vi "Configure.vi"(7 "Enum":enum16{"Read", "Write"}(ring), 11 "Port 4":refnum<vi>) -> (3 "Port 5":refnum<vi>)   [LabVIEW 2013]
uses:
  Control/Port.ctl
  Control/Buffer.vi
  <vilib>/Utility/config.llb/Read Key (String).vi
  <vilib>/Utility/config.llb/Read Key (I32).vi
  <vilib>/Utility/config.llb/Write Key (String).vi
  <vilib>/Utility/config.llb/NI_LVConfig.lvlib
panel:
  out "Boolean":bool
  out "s? t:f":string
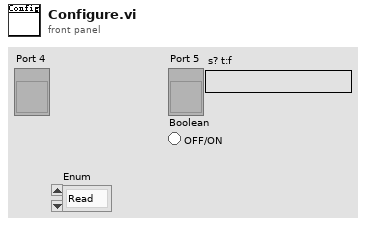
[diagram p1: front panel]
types:
  T1 = typedef "NI_LVConfig.lvlib/Config Data RefNum.ctl" = refnum<k1>
  T2 = typedef "Port.ctl" = cluster{"Multimeter":refnum<visa-resource-name>, "ACsource ":refnum<visa-resource-name>, "GEA":refnum<visa-resource-name>, "WT200":refnum<visa-resource-name>, "AutoScan":refnum<visa-resource-name>, "lines":tag, "MabeCOM":refnum<visa-resource-name>}
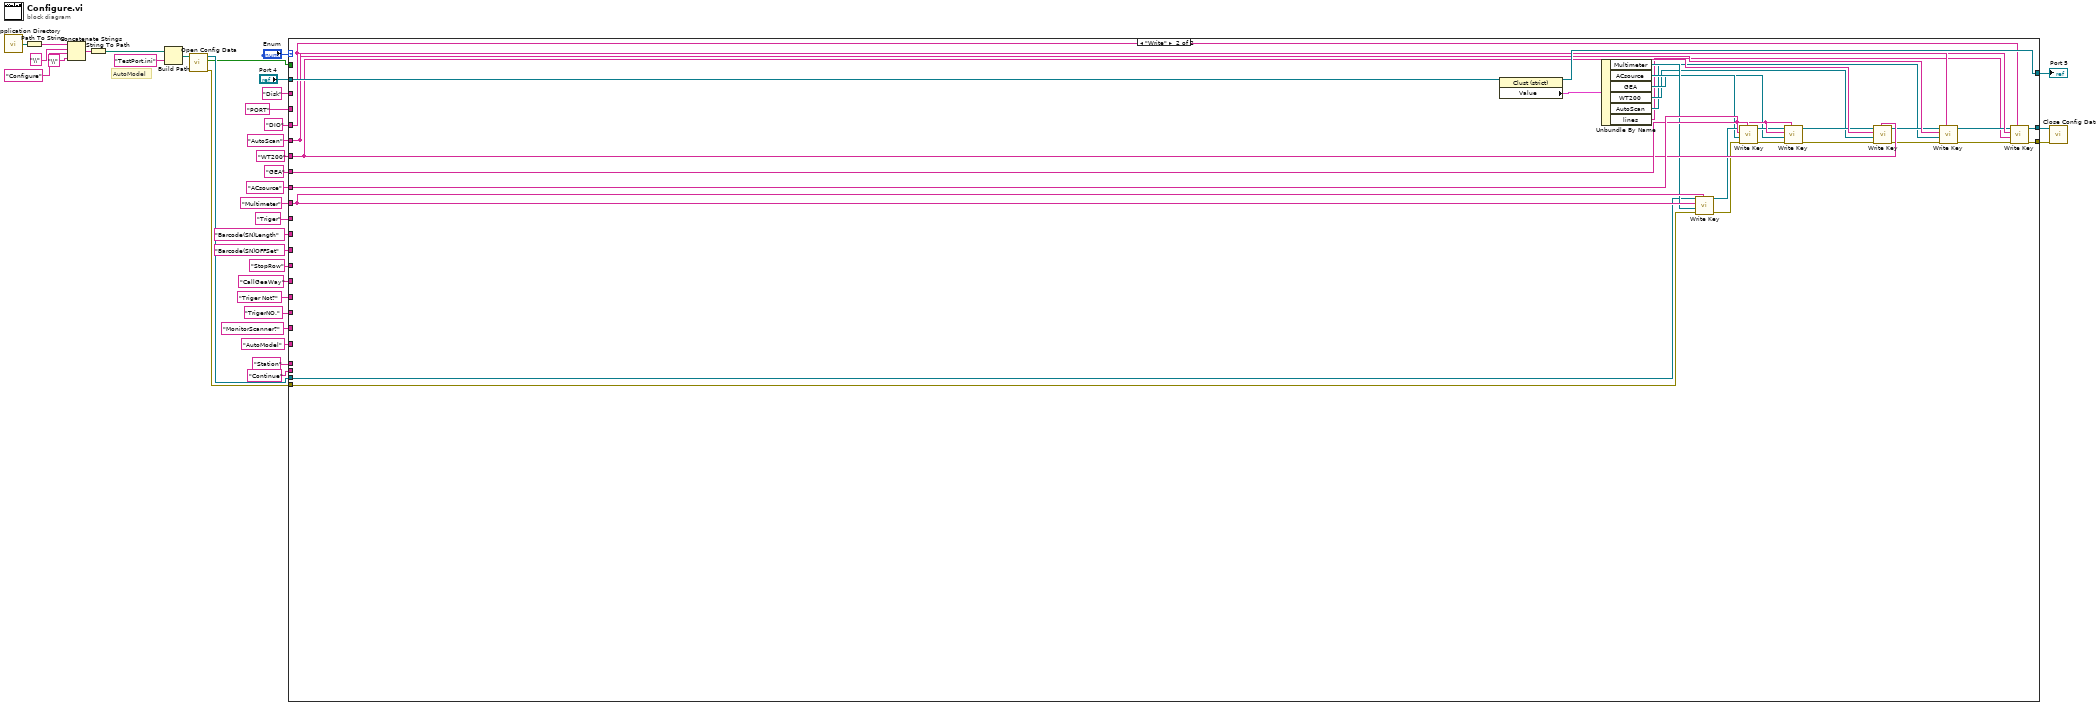
[diagram p0: block diagram]
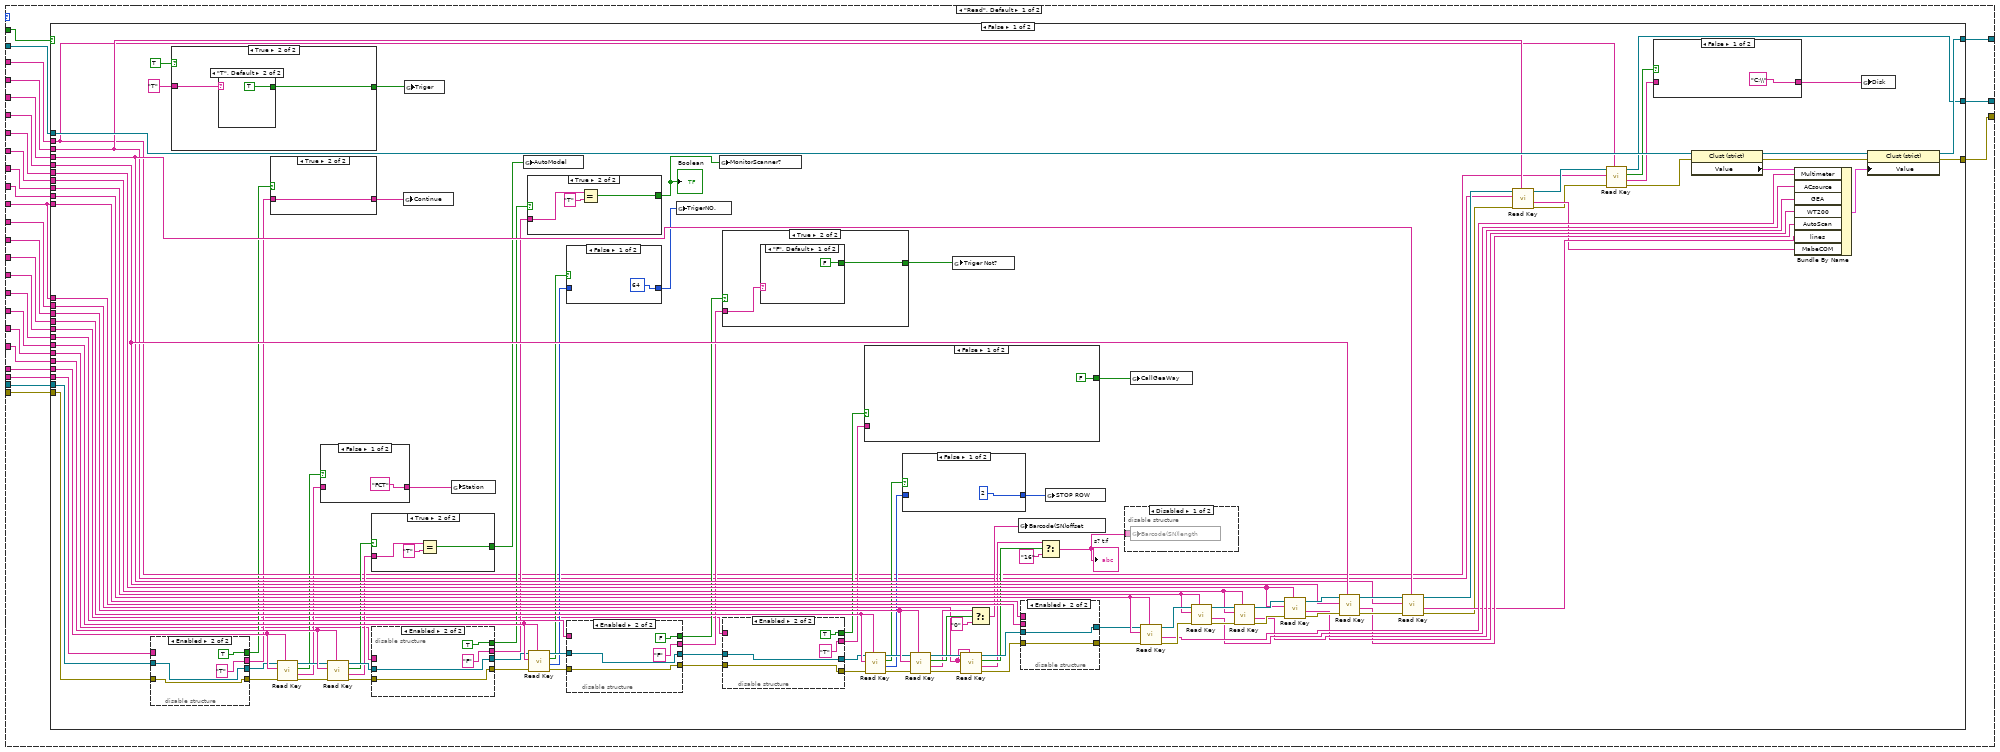
[diagram p2: hidden frame]
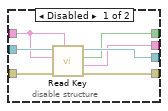
[diagram p4: hidden frame]
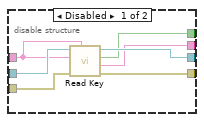
[diagram p5: hidden frame]
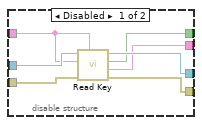
[diagram p6: hidden frame]
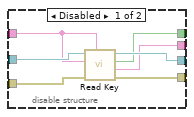
[diagram p7: hidden frame]
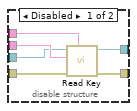
[diagram p8: hidden frame]
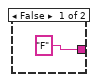
[diagram p9: hidden frame]
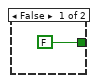
[diagram p12: hidden frame]
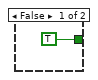
[diagram p13: hidden frame]
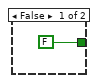
[diagram p14: hidden frame]
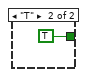
[diagram p15: hidden frame]
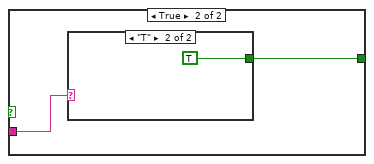
[diagram p17: hidden frame]
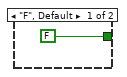
[diagram p18: hidden frame]
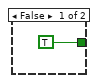
[diagram p20: hidden frame]
diagram:
  # "AutoModel"
  n1 = call <vilib>:"Application Directory.vi"() -> ("Application Directory"=w22:path)
  n2 = Path To String(path=w22) -> (string=w21:string)
  n3 = Concatenate Strings(w21, "\\" ("string"), "Configure" ("string"), "\\" ("string")) -> (w18:string)
  n4 = String To Path(string=w18) -> (path=w16:path)
  n5 = Build Path(base path=w16, name or relative path="TestPort.ini") -> (appended path=w34:path)
  n6 = call <vilib>:"Open Config Data.vi"("configuration file path"=w34) -> ("error out"=w32:errorcluster, "file created?"=w23:bool, "refnum"=w33:T1)  [unwired: 8 in]
  n7 = case shown="\"Write\"" "Enum" {
    tunnel: "Port 4" -> [w59 w292]
    tunnel: [w62 w291] -> w5
    tunnel: w33 -> [w61 w265]
    tunnel: w32 -> [w60 w264]
    tunnel: "Multimeter" ("section") -> [w56 w289]
    tunnel: "ACsource" ("section") -> [w55 w288]
    tunnel: "GEA" ("section") -> [w54 w287]
    tunnel: "WT200" ("section") -> [w53 w286]
    tunnel: "AutoScan" ("section") -> [w52 w285]
    tunnel: "DIO" ("section") -> [w51 w284]
    tunnel: [w57 w267] -> w25
    tunnel: [w58 w266] -> w24
    tunnel: w23 -> [w50 _]
    tunnel: "Triger" ("section") -> [w39 _]
    tunnel: "Barcode(SN)OFFSet" -> [w49 _]
    tunnel: "Barcode(SN)Length" -> [w37 _]
    tunnel: "StopRow" -> [w48 _]
    tunnel: "CallGeaWay" -> [w47 _]
    tunnel: "TrigerNO." -> [w46 _]
    tunnel: "Triger Not?" -> [w45 _]
    tunnel: "MonitorScanner?" ("section") -> [w38 _]
    tunnel: "AutoModel" -> [w44 _]
    tunnel: "PORT" -> [w43 _]
    tunnel: "Disk" -> [w42 _]
    tunnel: "Station" -> [w41 _]
    tunnel: "Continue" -> [w40 _]
    frame "Read", Default {
      n8 = case shown="False" w50 {
        tunnel: [w174 w263] -> w62
        tunnel: w61 -> [w72 w262]
        tunnel: w60 -> [w70 w261]
        tunnel: w59 -> [w173 w263]
        tunnel: [w148 w261] -> w58
        tunnel: [w85 w262] -> w57
        tunnel: w56 -> [w161 _]
        tunnel: w55 -> [w160 _]
        tunnel: w54 -> [w159 _]
        tunnel: w53 -> [w158 _]
        tunnel: w52 -> [w157 _]
        tunnel: w51 -> [w156 _]
        tunnel: w39 -> [w147 _]
        tunnel: w39 -> [w146 _]
        tunnel: w49 -> [w128 _]
        tunnel: w37 -> [w127 _]
        tunnel: w48 -> [w124 _]
        tunnel: w47 -> [w65 _]
        tunnel: w46 -> [w115 _]
        tunnel: w45 -> [w110 _]
        tunnel: w38 -> [w64 _]
        tunnel: w44 -> [w97 _]
        tunnel: w43 -> [w87 _]
        tunnel: w42 -> [w82 _]
        tunnel: w41 -> [w76 _]
        tunnel: w40 -> [w63 _]
        frame False {
          n9 = disable-structure shown="Enabled" {
            disable-tunnel: w72 -> [w182 w185]
            disable-tunnel: [w181 w185] -> w71
            disable-tunnel: w70 -> [w180 w186]
            disable-tunnel: [w179 w186] -> w69
            disable-tunnel: [w178 TRUE ("found?")] -> w68
            disable-tunnel: [w177 "T"] -> w67
            disable-tunnel: w63 -> [w176 _]
            frame Disabled {
              n10 = call-poly <vilib>:"Read Key.vi"("section"=w176, "error in (no error)"=w180, "key"=w176, "refnum"=w182) -> ("error out"=w179:errorcluster, "value"=w177:string, "found?"=w178:bool, "refnum out"=w181:T1)  [unwired: 4 in]
            }
            frame Enabled {
            }
          }
          n11 = case shown="True" TRUE ("found?") {
            tunnel: "T" ("value") -> [_ w258]
            tunnel: [TRUE w257] -> w141
            frame False {
            }
            frame True {
              n12 = case shown="\"T\", Default" w258 {
                tunnel: [FALSE TRUE] -> w257
                frame "F" {
                }
                frame "T", Default {
                }
              }
            }
          }
          n13 = case shown="True" w68 {
            tunnel: w67 -> [_ w229]
            tunnel: ["F" ("value") w229] -> w66
            frame False {
            }
            frame True {
            }
          }
          n14 = call-poly <vilib>:"Read Key.vi"("section"=w76, "error in (no error)"=w69, "key"=w76, "refnum"=w71) -> ("error out"=w77:errorcluster, "value"=w75:string, "found?"=w74:bool, "refnum out"=w78:T1)  [unwired: 4 in]
          n15 = case shown="False" w74 {
            tunnel: w75 -> [_ w231]
            tunnel: ["FCT" ("value") w231] -> w73
            frame False {
            }
            frame True {
            }
          }
          n16 = call-poly <vilib>:"Read Key.vi"("section"=w97, "error in (no error)"=w77, "key"=w97, "refnum"=w78) -> ("error out"=w95:errorcluster, "value"=w94:string, "found?"=w93:bool, "refnum out"=w96:T1)  [unwired: 4 in]
          n17 = case shown="True" w93 {
            tunnel: [FALSE w235] -> w98
            tunnel: w94 -> [_ w237]
            frame False {
            }
            frame True {
              n18 = Equal?(x=w237, y="T") -> (x = y?=w235:bool)
            }
          }
          n19 = disable-structure shown="Enabled" {
            disable-tunnel: [w193 w196] -> w103
            disable-tunnel: [w192 w197] -> w102
            disable-tunnel: [w191 "F"] -> w100
            disable-tunnel: [w190 TRUE ("found?")] -> w99
            disable-tunnel: w96 -> [w189 w196]
            disable-tunnel: w95 -> [w188 w197]
            disable-tunnel: w64 -> [w187 _]
            frame Disabled {
              n20 = call-poly <vilib>:"Read Key.vi"("section"=w187, "error in (no error)"=w188, "key"=w187, "refnum"=w189) -> ("error out"=w192:errorcluster, "value"=w191:string, "found?"=w190:bool, "refnum out"=w193:T1)  [unwired: 4 in]
            }
            frame Enabled {
            }
          }
          n21 = global write "Buffer.vi" "Continue"(w66) -> ()
          n22 = global write "Buffer.vi" "Triger"(w141) -> ()
          n23 = global write "Buffer.vi" "Station"(w73) -> ()
          n24 = global write "Buffer.vi" "AutoModel"(w98) -> ()
          n25 = case shown="True" w99 {
            tunnel: [TRUE w239] -> w101
            tunnel: w100 -> [_ w241]
            frame False {
            }
            frame True {
              n26 = Equal?(x=w241, y="T") -> (x = y?=w239:bool)
            }
          }
          "Boolean" <- w101
          n27 = call-poly <vilib>:"Read Key.vi"("section"=w115, "error in (no error)"=w102, "key"=w115, "refnum"=w103) -> ("error out"=w114:errorcluster, "value"=w108:i32, "found?"=w109:bool, "refnum out"=w113:T1)  [unwired: 4 in]
          n28 = case shown="False" w109 {
            tunnel: w108 -> [_ w248]
            tunnel: [64 ("value") w248] -> w107
            frame False {
            }
            frame True {
            }
          }
          n29 = disable-structure shown="Enabled" {
            disable-tunnel: w114 -> [w215 w219]
            disable-tunnel: w113 -> [w214 w218]
            disable-tunnel: [w213 w218] -> w112
            disable-tunnel: [w212 w219] -> w111
            disable-tunnel: w110 -> [w211 _]
            disable-tunnel: [w210 FALSE] -> w106
            disable-tunnel: [w209 "F"] -> w105
            frame Disabled {
              n30 = call-poly <vilib>:"Read Key.vi"("section"=w211, "error in (no error)"=w215, "key"=w211, "refnum"=w214) -> ("error out"=w212:errorcluster, "value"=w209:string, "found?"=w210:bool, "refnum out"=w213:T1)  [unwired: 4 in]
            }
            frame Enabled {
            }
          }
          n31 = global write "Buffer.vi" "TrigerNO."(w107) -> ()
          n32 = global write "Buffer.vi" "MonitorScanner?"(w101) -> ()
          n33 = case shown="True" w106 {
            tunnel: w105 -> [_ w244]
            tunnel: [FALSE ("value") w243] -> w104
            frame False {
            }
            frame True {
              n34 = case shown="\"F\", Default" w244 {
                tunnel: [FALSE TRUE] -> w243
                frame "F", Default {
                }
                frame "T" {
                }
              }
            }
          }
          n35 = disable-structure shown="Enabled" {
            disable-tunnel: [w204 w207] -> w120
            disable-tunnel: [w203 w208] -> w119
            disable-tunnel: [w202 "T"] -> w118
            disable-tunnel: [w201 TRUE] -> w116
            disable-tunnel: w112 -> [w200 w207]
            disable-tunnel: w111 -> [w199 w208]
            disable-tunnel: w65 -> [w198 _]
            frame Disabled {
              n36 = call-poly <vilib>:"Read Key.vi"("section"=w198, "error in (no error)"=w199, "key"=w198, "refnum"=w200) -> ("error out"=w203:errorcluster, "value"=w202:string, "found?"=w201:bool, "refnum out"=w204:T1)  [unwired: 4 in]
            }
            frame Enabled {
            }
          }
          n37 = case shown="False" w116 {
            tunnel: w118 -> [_ w251]
            tunnel: [FALSE w250] -> w117
            frame False {
            }
            frame True {
              n38 = case shown="\"T\"" w251 {
                tunnel: [FALSE TRUE] -> w250
                frame "F", Default {
                }
                frame "T" {
                }
              }
            }
          }
          n39 = call-poly <vilib>:"Read Key.vi"("section"=w124, "error in (no error)"=w119, "key"=w124, "refnum"=w120) -> ("error out"=w125:errorcluster, "value"=w122:i32, "found?"=w123:bool, "refnum out"=w126:T1)  [unwired: 4 in]
          n40 = case shown="False" w123 {
            tunnel: w122 -> [_ w255]
            tunnel: [2 ("value") w255] -> w121
            frame False {
            }
            frame True {
            }
          }
          n41 = call-poly <vilib>:"Read Key.vi"("section"=w128, "error in (no error)"=w125, "key"=w128, "refnum"=w126) -> ("error out"=w138:errorcluster, "value"=w134:string, "found?"=w136:bool, "refnum out"=w140:T1)  [unwired: 4 in]
          n42 = global write "Buffer.vi" "Triger Not?"(w104) -> ()
          n43 = call-poly <vilib>:"Read Key.vi"("section"=w127, "error in (no error)"=w138, "key"=w127, "refnum"=w140) -> ("error out"=w137:errorcluster, "value"=w130:string, "found?"=w131:bool, "refnum out"=w139:T1)  [unwired: 4 in]
          n44 = Select(t=w134, s=w136, f="0") -> (s? t:f=w135:string)
          n45 = global write "Buffer.vi" "Barcode(SN)offset"(w135) -> ()
          n46 = disable-structure shown="Enabled" {
            disable-tunnel: w147 -> [w225 _]
            disable-tunnel: w146 -> [w224 _]
            disable-tunnel: [w223 w226] -> w145
            disable-tunnel: [w222 w227] -> w144
            disable-tunnel: w139 -> [w221 w226]
            disable-tunnel: w137 -> [w220 w227]
            frame Disabled {
              n47 = call-poly <vilib>:"Read Key.vi"("section"=w225, "error in (no error)"=w220, "key"=w224, "refnum"=w221) -> ("error out"=w222:errorcluster, "refnum out"=w223:T1)  [unwired: 4 in, 2 out]
            }
            frame Enabled {
            }
          }
          n48 = Select(t=w130, s=w131, f="16") -> (s? t:f=w129:string)
          "s? t:f" <- w129
          n49 = global write "Buffer.vi" "STOP ROW"(w121) -> ()
          n50 = disable-structure shown="Disabled" {
            disable-tunnel: w129 -> [w175 _]
            frame Disabled {
              n51 = global write "Buffer.vi" "Barcode(SN)length"(w175) -> ()
            }
            frame Enabled {
            }
          }
          n52 = global write "Buffer.vi" "CallGeaWay"(w117) -> ()
          n53 = call-poly <vilib>:"Read Key.vi"("section"=w161, "error in (no error)"=w144, "key"=w161, "refnum"=w145) -> ("error out"=w170:errorcluster, "value"=w155:string, "refnum out"=w171:T1)  [unwired: 4 in, 1 out]
          n54 = call-poly <vilib>:"Read Key.vi"("section"=w160, "error in (no error)"=w170, "key"=w160, "refnum"=w171) -> ("error out"=w162:errorcluster, "value"=w154:string, "refnum out"=w169:T1)  [unwired: 4 in, 1 out]
          n55 = call-poly <vilib>:"Read Key.vi"("section"=w159, "error in (no error)"=w162, "key"=w159, "refnum"=w169) -> ("error out"=w163:errorcluster, "value"=w153:string, "refnum out"=w168:T1)  [unwired: 4 in, 1 out]
          n56 = call-poly <vilib>:"Read Key.vi"("section"=w158, "error in (no error)"=w163, "key"=w158, "refnum"=w168) -> ("error out"=w164:errorcluster, "value"=w152:string, "refnum out"=w167:T1)  [unwired: 4 in, 1 out]
          n57 = call-poly <vilib>:"Read Key.vi"("section"=w157, "error in (no error)"=w164, "key"=w157, "refnum"=w167) -> ("error out"=w165:errorcluster, "value"=w151:string, "refnum out"=w166:T1)  [unwired: 4 in, 1 out]
          n58 = call-poly <vilib>:"Read Key.vi"("section"=w156, "error in (no error)"=w165, "key"=w156, "refnum"=w166) -> ("error out"=w89:errorcluster, "value"=w150:string, "refnum out"=w88:T1)  [unwired: 4 in, 1 out]
          n59 = call-poly <vilib>:"Read Key.vi"("section"=w87, "error in (no error)"=w89, "key"=w87, "refnum"=w88) -> ("error out"=w84:errorcluster, "value"=w90:string, "refnum out"=w86:T1)  [unwired: 4 in, 1 out]
          n60 = call-poly <vilib>:"Read Key.vi"("section"=w82, "error in (no error)"=w84, "key"=w82, "refnum"=w86) -> ("error out"=w83:errorcluster, "value"=w81:string, "found?"=w80:bool, "refnum out"=w85:T1)  [unwired: 4 in]
          n61 = case shown="False" w80 {
            tunnel: w81 -> [_ w233]
            tunnel: ["C:\\" ("value") w233] -> w79
            frame False {
            }
            frame True {
            }
          }
          n62 = property class="Clust (strict)"(reference=w173, error in=w83) -> (reference out=w172:refnum<vi>, error out=w149:errorcluster, "Value"=w92:T2)
          n63 = Bundle By Name(cluster=w92, "Multimeter"=w155, "ACsource"=w154, "GEA"=w153, "WT200"=w152, "AutoScan"=w151, "lines"=w150, "MabeCOM"=w90) -> (w91:T2)
          n64 = global write "Buffer.vi" "Disk"(w79) -> ()
          n65 = property class="Clust (strict)"(reference=w172, error in=w149, "Value"=w91) -> (reference out=w174:refnum<vi>, error out=w148:errorcluster)
        }
        frame True {
        }
      }
    }
    frame "Write" {
      n66 = property class="Clust (strict)"(reference=w292) -> (reference out=w291:refnum<vi>, "Value"=w290:T2)  [unwired: 1 in, 1 out]
      n67 = Unbundle By Name(w290) -> ("Multimeter"=w273:refnum<visa-resource-name>, "ACsource"=w272:refnum<visa-resource-name>, "GEA"=w271:refnum<visa-resource-name>, "WT200"=w270:refnum<visa-resource-name>, "AutoScan"=w269:refnum<visa-resource-name>, "lines"=w268:tag)
      n68 = call-poly <vilib>:"Write Key.vi"("section"=w289, "error in (no error)"=w264, "value"=w273, "key"=w289, "refnum"=w265) -> ("error out"=w274:errorcluster, "refnum out"=w283:T1)  [unwired: 4 in, 1 out]
      n69 = call-poly <vilib>:"Write Key.vi"("section"=w288, "error in (no error)"=w274, "value"=w272, "key"=w288, "refnum"=w283) -> ("error out"=w275:errorcluster, "refnum out"=w282:T1)  [unwired: 4 in, 1 out]
      n70 = call-poly <vilib>:"Write Key.vi"("section"=w287, "error in (no error)"=w275, "value"=w271, "key"=w287, "refnum"=w282) -> ("error out"=w276:errorcluster, "refnum out"=w281:T1)  [unwired: 4 in, 1 out]
      n71 = call-poly <vilib>:"Write Key.vi"("section"=w286, "error in (no error)"=w276, "value"=w270, "key"=w286, "refnum"=w281) -> ("error out"=w277:errorcluster, "refnum out"=w280:T1)  [unwired: 4 in, 1 out]
      n72 = call-poly <vilib>:"Write Key.vi"("section"=w285, "error in (no error)"=w277, "value"=w269, "key"=w285, "refnum"=w280) -> ("error out"=w278:errorcluster, "refnum out"=w279:T1)  [unwired: 4 in, 1 out]
      n73 = call-poly <vilib>:"Write Key.vi"("section"=w284, "error in (no error)"=w278, "value"=w268, "key"=w284, "refnum"=w279) -> ("error out"=w266:errorcluster, "refnum out"=w267:T1)  [unwired: 4 in, 1 out]
    }
  }
  "Port 5" <- w5
  n74 = call <vilib>:"Close Config Data.vi"("error in (no error)"=w24, "refnum"=w25) -> ()  [unwired: 8 in, 2 out]
